vi "Get SMO Name.vi"(8 "error in (no error)":errorcluster, 11 "FP-TC-Shared in":refnum<class "FP-TC-Shared.lvclass">) -> (0 "error out":errorcluster, 2 "SMO Name":string, 3 "FP-TC-Shared out":refnum<class "FP-TC-Shared.lvclass">)   [LabVIEW 2019, in "FP-TC-Shared.lvclass"]
uses:
  FP-TC-Shared.lvclass
  C:/Program Files (x86)/National Instruments/LabVIEW 2019/user.lib/LevyLab/Instrument Framework/SMOs/Instrument/Instrument.lvclass
  FP-TC-Shared.lvclass/FP-TC-Shared.ctl
  <userlib>/LevyLab/Instrument Framework/Instrument Types/Cryostat/Instrument.Cryostat.lvclass
  <userlib>/LevyLab/Instrument Framework/SMOs/Instrument/Instrument.lvclass
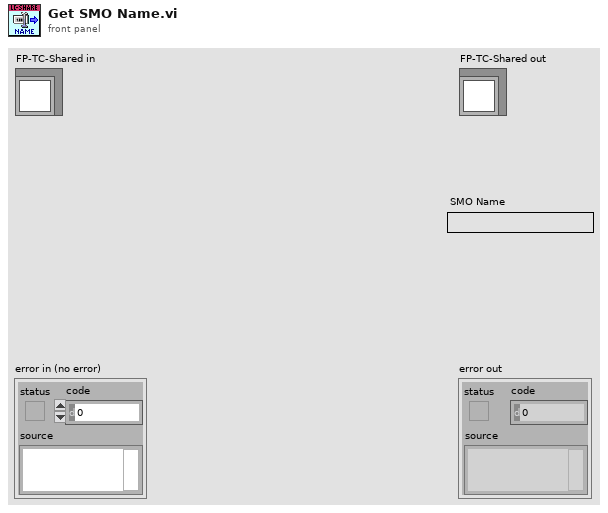
[diagram p1: front panel]
types:
  T1 = typedef "FP-TC-Shared.lvclass/LC Type--Enum.ctl" = enum16{"CF.TC", "CF.TC.Z", "CF.FP", "MNK.TC", "MNK.TC.Z", "MNK.FP"}
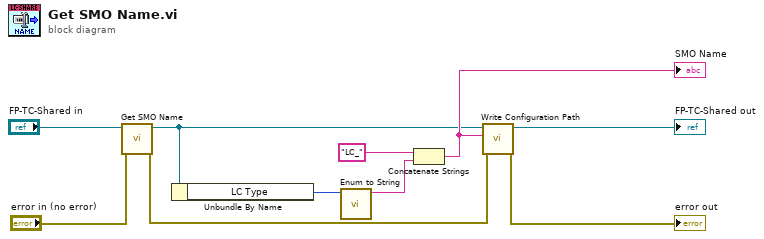
[diagram p0: block diagram]
diagram:
  n1 = call-parent "Get SMO Name.vi"("error in (no error)"="error in (no error)", "Instrument in"="FP-TC-Shared in") -> ("error out"=w4:errorcluster, "Instrument out"=w3:refnum<class "FP-TC-Shared.lvclass">)  [unwired: 7 in, 1 out]
  n2 = Unbundle By Name(w3) -> ("LC Type"=w2:T1)
  n3 = call <userlib>:"Enum to String.vi"("Command"=w2) -> ("Command"=w1:string)  [unwired: 9 in, 1 out]
  n4 = Concatenate Strings("LC_" ("SMO Name"), w1) -> (w6:string)
  "SMO Name" <- w6
  n5 = call <userlib>:"Write Configuration Path.vi"("error in (no error)"=w4, "name or relative path"=w6, "Instrument in"=w3) -> ("error out"=→"error out":errorcluster, "Instrument out"=→"FP-TC-Shared out":refnum<class "FP-TC-Shared.lvclass">)  [unwired: 7 in]
